vi "create_full_endpoint.vi"(8 "error in (no error)":errorcluster, 11 "llm_openai_embedding in":refnum<class "llm_gemini_embedding.lvclass">) -> (0 "error out":errorcluster, 2 "endpoint":string, 3 "llm_openai_embedding out":refnum<class "llm_gemini_embedding.lvclass">)   [LabVIEW 2020, in "llm_gemini_embedding.lvclass"]
uses:
  llm_gemini_embedding.lvclass
  llm_gemini_embedding.lvclass/llm_gemini_embedding.ctl
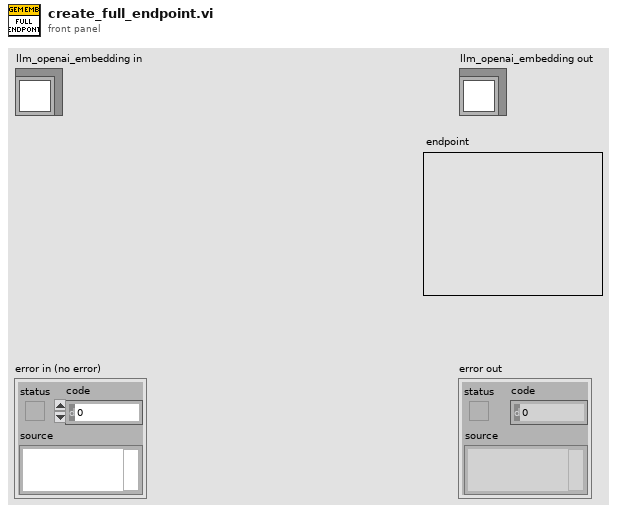
[diagram p1: front panel]
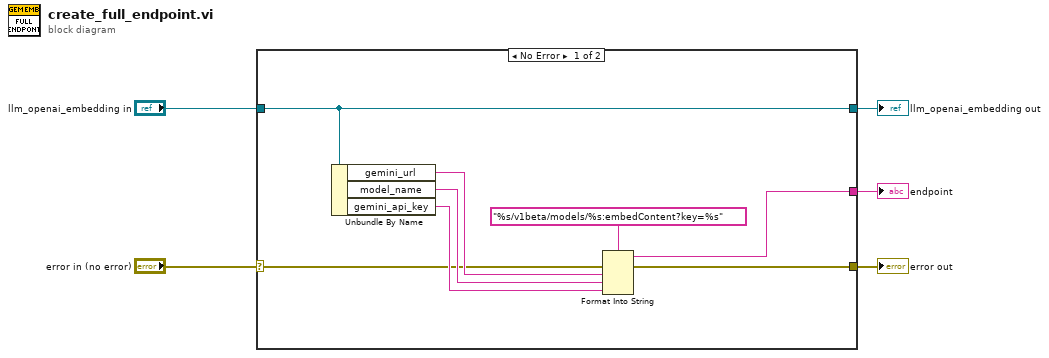
[diagram p0: block diagram]
diagram:
  n1 = case shown="No Error" "error in (no error)" {
    selector: "error in (no error)" -> [w7 w15]
    tunnel: [w6 w15] -> w4
    tunnel: [w9 w14] -> w2
    tunnel: "llm_openai_embedding in" -> [w9 w14]
    tunnel: [w8 _] -> w1
    frame No Error {
      n2 = Unbundle By Name(w9) -> ("gemini_url"=w13:string, "model_name"=w12:string, "gemini_api_key"=w11:string)
      n3 = Format Into String(format string="%s/v1beta/models/%s:embedContent?key=%s", error in=w7, w13, w12, w11) -> (resulting string=w8:string, error out=w6:errorcluster)  [unwired: 1 in]
    }
    frame Error {
    }
  }
  "error out" <- w4
  "llm_openai_embedding out" <- w2
  "endpoint" <- w1
